vi "计算温度值.vi"(9 "数值L":u8, 10 "数值H":u8) -> (2 "温度":dbl)   [LabVIEW 2013]
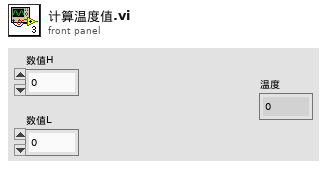
[diagram p1: front panel]
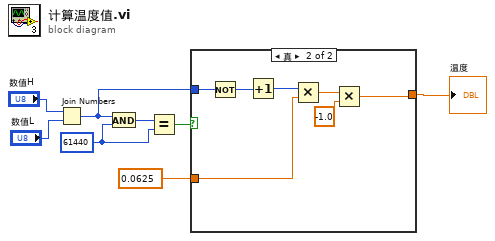
[diagram p0: block diagram]
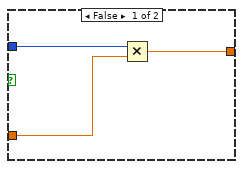
[diagram p2: hidden frame]
diagram:
  w5 = u16 61440 ("y")
  n1 = Join Numbers(hi="数值H", lo="数值L") -> ((hi.lo)=w3:u16)
  n2 = And(x=w3, y=w5) -> (x .and. y?=w6:u16)
  n3 = Equal?(x=w6, y=w5) -> (x = y?=w4:bool)
  n4 = case shown="真" w4 {
    tunnel: w3 -> [w10 w17]
    tunnel: [w9 w12] -> w1
    tunnel: 0.0625 ("y") -> [w11 w15]
    frame False {
      n5 = Multiply(x=w10, y=w11) -> (x*y=w9:dbl)
    }
    frame True {
      n6 = Not(x=w17) -> (.not. x?=w18:u16)
      n7 = Increment(x=w18) -> (x+1=w16:u16)
      n8 = Multiply(x=w16, y=w15) -> (x*y=w14:dbl)
      n9 = Multiply(x=w14, y=-1.0) -> (x*y=w12:dbl)
    }
  }
  "温度" <- w1
